vi "LvMPDC_SUB_DirScan.vi"(8 "error in (no error)":errorcluster, 10 "dir path":path, 11 "Connect ID":refnum<k5>) -> (0 "error out":errorcluster, 1 "file info[]":T2(array[cluster]) {"MusicInfo"."time" format="%<%H:%M:%S%3u>t"}, 3 "Connect ID out":refnum<k5>)   [LabVIEW 2012]
uses:
  LvMPDC_Typdef_MusicInfo.ctl
panel:
  # "LvMPDC:: DirScan - 再帰で全フォルダスキャン クローン共有による再入を有効にしています。"
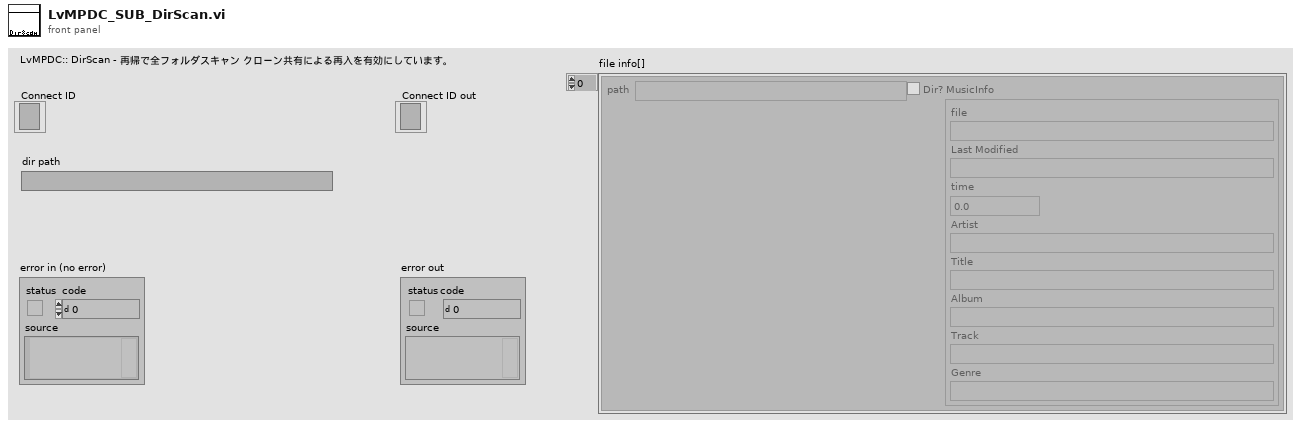
[diagram p1: front panel]
types:
  T1 = typedef "LvMPDC_Typdef_MusicInfo.ctl" = cluster{"file":string, "Last Modified":string, "time":dbl, "Artist":string, "Title":string, "Album":string, "Track":string, "Genre":string}
  T2 = cluster{"path":path, "Dir?":bool, "MusicInfo":T1}[]
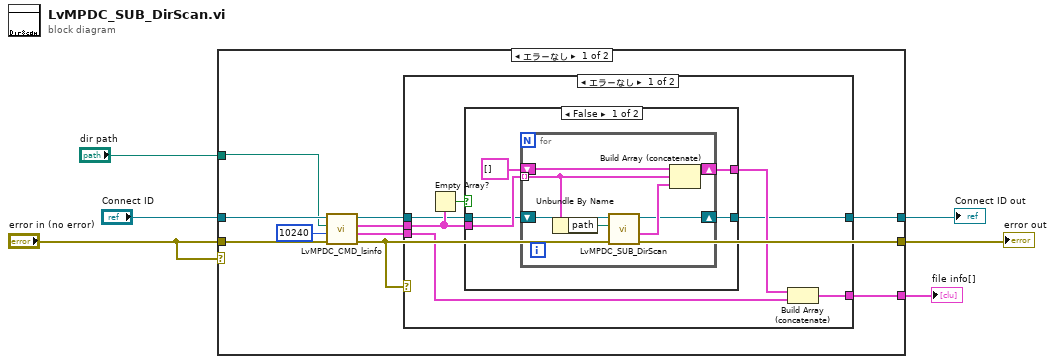
[diagram p0: block diagram]
diagram:
  n1 = case shown="エラーなし" "error in (no error)" {
    tunnel: "Connect ID" -> [w16 w39]
    tunnel: "error in (no error)" -> [w15 w38]
    tunnel: [w7 w39] -> w5
    tunnel: [w12 w38] -> w4
    tunnel: "dir path" -> [w13 _]
    tunnel: [w9 _] -> w1
    frame No Error {
      n2 = call "LvMPDC_CMD_lsinfo.vi"("error in (no error)"=w15, "ReadBytes"=10240, "filepath"=w13, "Connect ID"=w16) -> ("error out"=w12:errorcluster, "file info[]"=w10:T2, "folder info[]"=w11:T2, "Connect ID out"=w8:refnum<k5>)  [unwired: 4 in]
      n3 = case shown="エラーなし" w12 {
        tunnel: w11 -> [w21 _]
        tunnel: w10 -> [w20 _]
        tunnel: [w22 _] -> w9
        tunnel: w8 -> [w18 w37]
        tunnel: [w17 w37] -> w7
        frame No Error {
          n4 = Empty Array?(array=w21) -> (empty?=w23:bool)
          n5 = case shown="FALSE" w23 {
            tunnel: w21 -> [w28 _]
            tunnel: [w26 _] -> w19
            tunnel: w18 -> [w25 w36]
            tunnel: [w24 w36] -> w17
            frame False {
              n6 = for {
                tunnel: w28 -> [w32] mode=indexing
                shift-right: [w35] -> w26
                shift-left: T2 [] -> [w34]
                shift-right: [w29] -> w24
                shift-left: w25 -> [w30]
                n7 = Unbundle By Name(w32) -> ("path"=w31:path)
                n8 = call "LvMPDC_SUB_DirScan.vi"("dir path"=w31, "Connect ID"=w30) -> ("file info[]"=w33:T2, "Connect ID out"=w29:refnum<k5>)  [unwired: 7 in, 1 out]
                n9 = Build Array (concatenate)(w34, w32, w33) -> (w35:T2)
              }
            }
            frame True {
            }
          }
          n10 = Build Array (concatenate)(w19, w20) -> (w22:T2)
        }
        frame Error {
        }
      }
    }
    frame Error {
    }
  }
  "Connect ID out" <- w5
  "error out" <- w4
  "file info[]" <- w1
